vi "velosterpaser384.vi"(0 "roll":dbl=0.5000000000000001, 1 "pitch":dbl=-6.0, 2 "heading":dbl=1.2, 3 "dX":dbl=-0.009999999999999997, 4 "dY":dbl=1.287, 5 "dZ":dbl=1.6, 7 "Velodyne":T1(ring)=enum."Velodyne 64") -> (17 "pos_velo":dbl[](array[numeric]))   [LabVIEW 2015]
uses:
  G_LCM.vi
  G_SEN.vi
  <vilib>/Analysis/Matrix/Numeric/Conversions/Array To Matrix - RA2.vi
  <vilib>/Analysis/Matrix/Numeric/Multiply/Multiply - RM,RM.vi
  <vilib>/Analysis/Matrix/NI_Matrix.lvlib
panel:
  out "idx":i32[](array[numeric])
  out "Array":i32[](array[numeric])
  out "deleted portion":dbl[][](array[numeric])
  out "transposed array":dbl[][](array[numeric])
  out "o":dbl[](array[numeric])
  out "V":dbl[](array[numeric])
  out "R":dbl[](array[numeric])
  in  "PLOT":T1(ring)=enum."Velodyne 64"
  out "error out":errorcluster
  out "XY Graph 2":cluster{"X":dbl, "Y":dbl}[](graph)
  out "d":dbl[](array[numeric])
  in  "thresh":dbl
  out "i":u8[](array[numeric])
  out "Z":dbl[](array[numeric])
  out "Y":dbl[](array[numeric])
  out "X":dbl[](array[numeric])
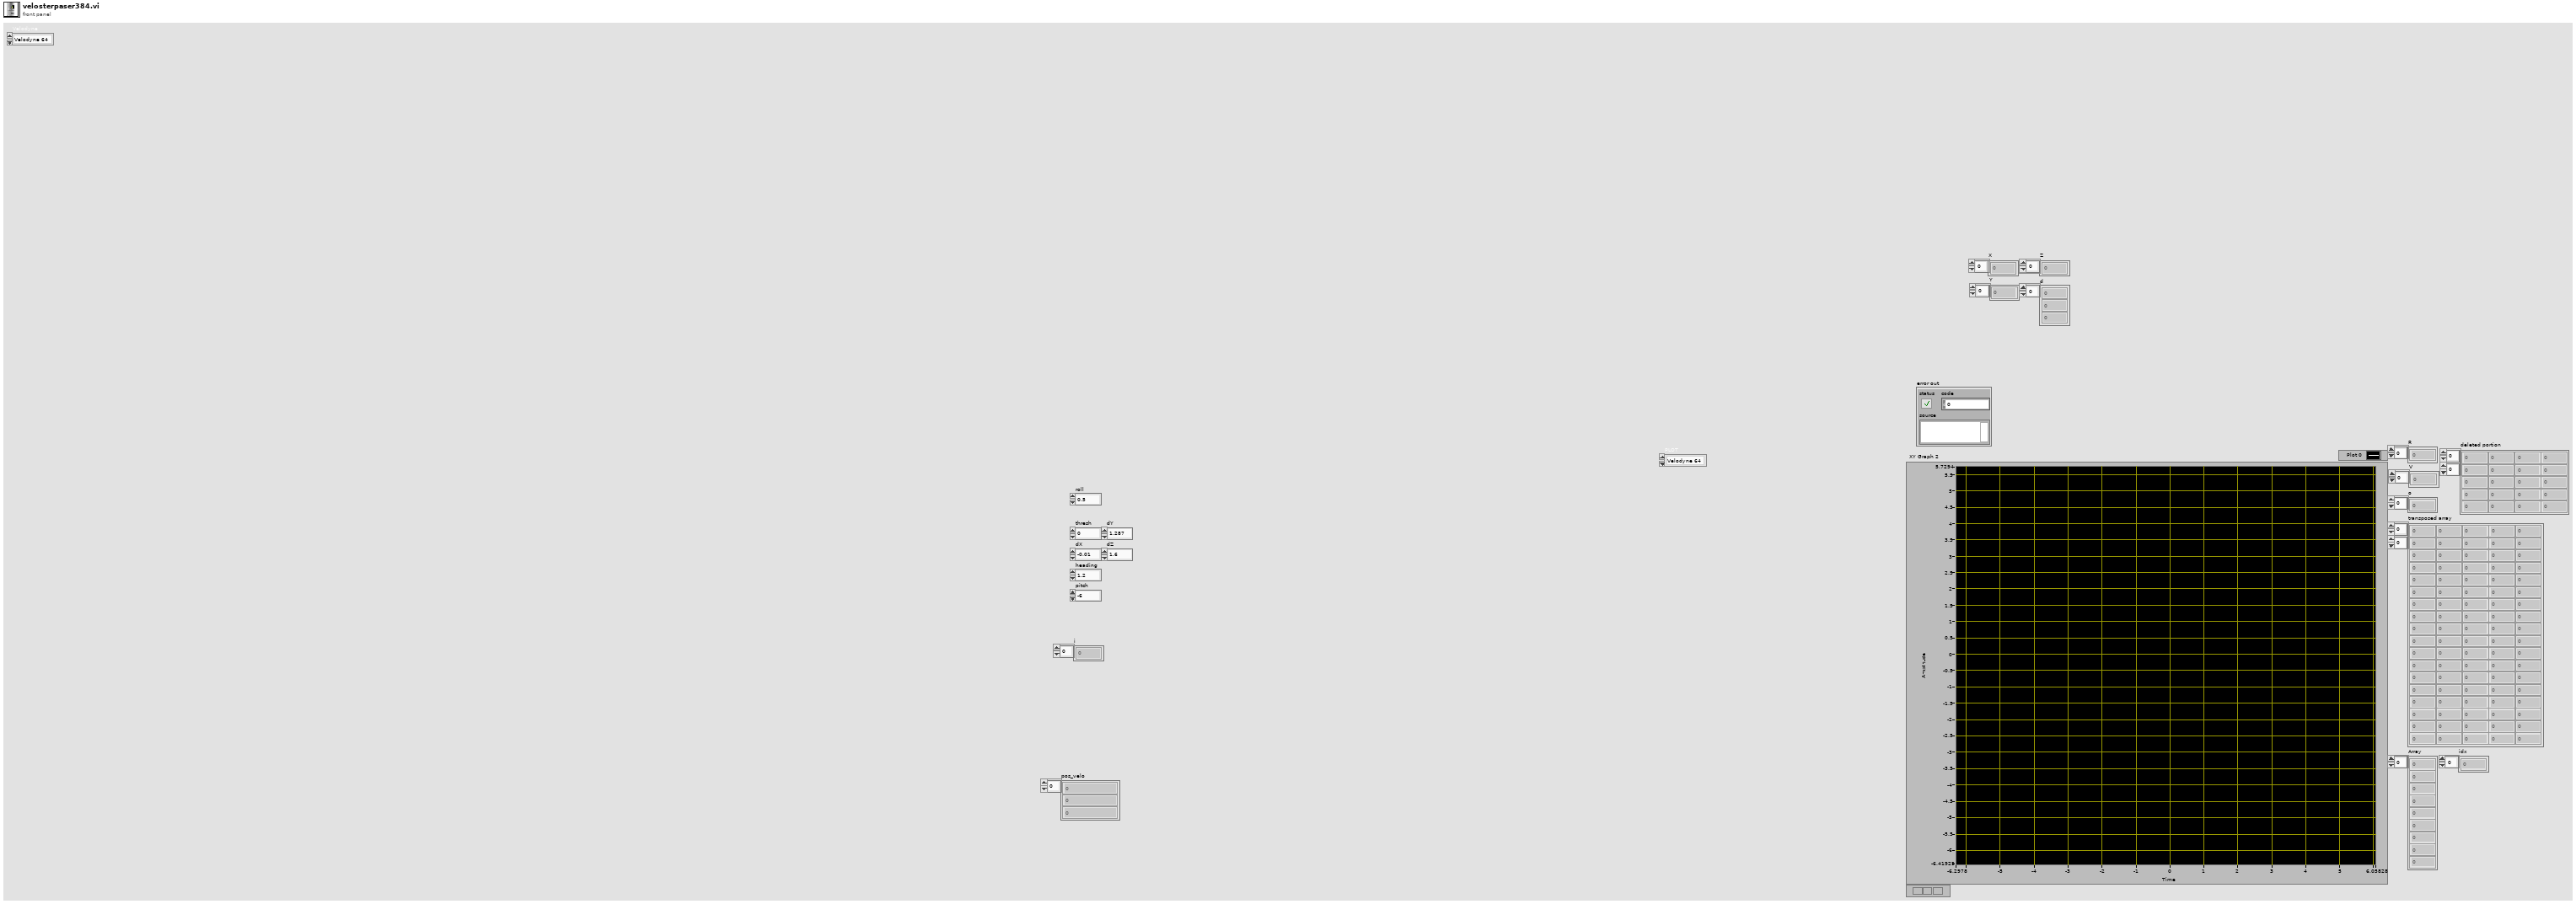
[diagram p1: front panel]
types:
  T1 = enum16{"Velodyne 16", "Velodyne 32", "Velodyne 64"}
  T2 = cluster{"hash":i64, "sys time":i64, "Timestamp":u32, "Rot_ang":dbl[], "Ver_ang":dbl[], "Dist":dbl[], "Ver_off":dbl[], "Intensity":u8[], "pos x":dbl, "pos y":dbl, "Heading":dbl}
  T3 = typedef "NI_Matrix.lvlib/RealMatrix.ctl" = dbl[][]
  T4 = cluster{i16, dbl, dbl, dbl, "Rotational position":dbl, "element":u8}[]
  T5 = cluster{dbl, i32, dbl, "Rotational position":dbl, dbl, "element":u8}[]
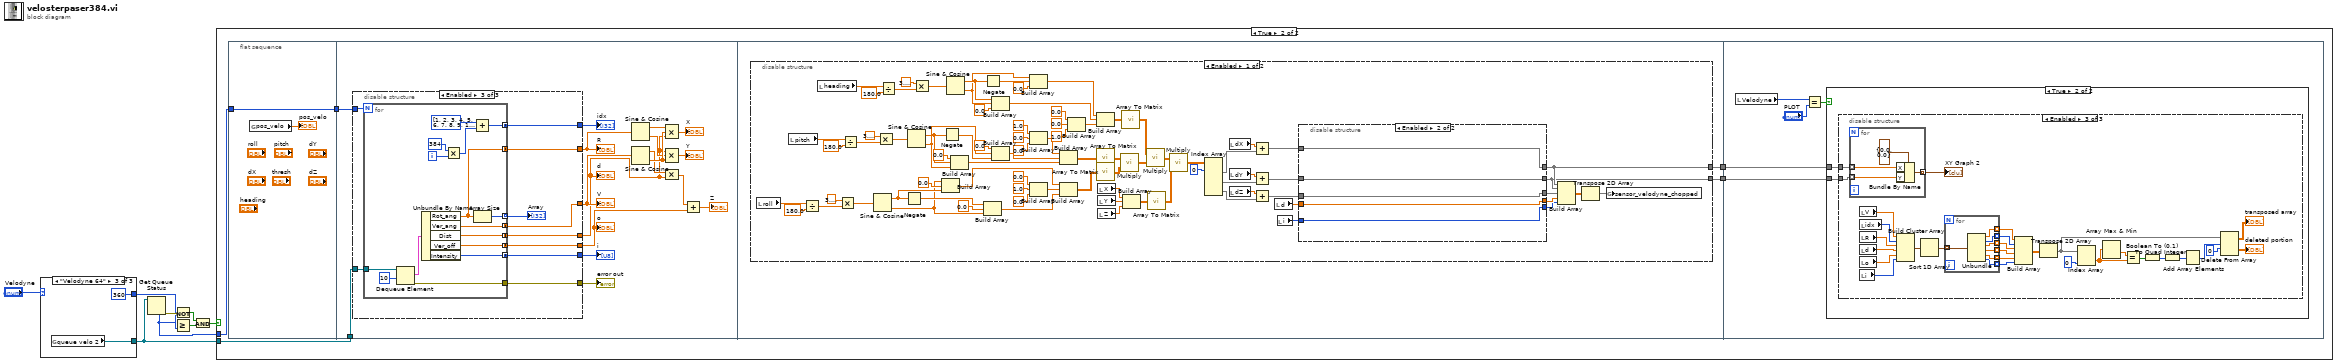
[diagram p0: block diagram]
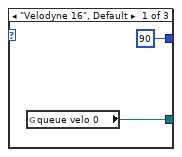
[diagram p2: hidden frame]
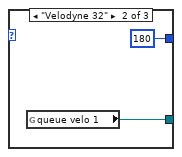
[diagram p3: hidden frame]
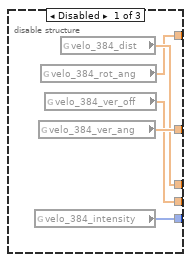
[diagram p5: hidden frame]
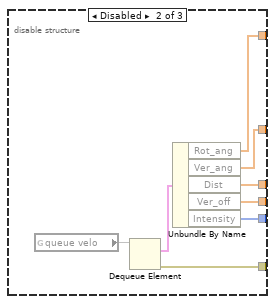
[diagram p6: hidden frame]
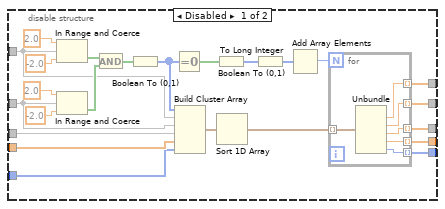
[diagram p7: hidden frame]
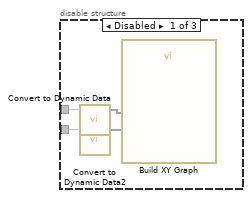
[diagram p10: hidden frame]
diagram:
  n1 = case shown="\"Velodyne 64\"" "Velodyne" {
    tunnel: [90 ("Numeric") 180 360 ("Numeric")] -> w5
    tunnel: [w9 w11 w13] -> w1
    frame "Velodyne 16", Default {
      n2 = global read "G_LCM.vi" "queue velo 0"() -> (w9:refnum<queue>)
    }
    frame "Velodyne 32" {
      n3 = global read "G_LCM.vi" "queue velo 1"() -> (w11:refnum<queue>)
    }
    frame "Velodyne 64" {
      n4 = global read "G_LCM.vi" "queue velo 2"() -> (w13:refnum<queue>)
    }
  }
  n5 = Get Queue Status(queue=w1) -> (error out=w7:errorcluster, # elements in queue=w2:i32)  [unwired: 2 in, 6 out]
  n6 = Not(x=w7) -> (.not. x?=w6:bool)
  n7 = Greater Or Equal?(x=w2, y=w5) -> (x >= y?=w8:bool)
  n8 = And(x=w6, y=w8) -> (x .and. y?=w4:bool)
  n9 = case shown="True" w4 {
    tunnel: w2 -> [_ w16]
    tunnel: w1 -> [_ w15]
    frame False {
    }
    frame True {
      n10 = flat-sequence {
        tunnel: [w20] -> w17
        tunnel: w16 -> [w20]
        tunnel: w17 -> [w24]
        tunnel: w15 -> [w23]
        tunnel: [w78] -> w19
        tunnel: [w77] -> w18
        tunnel: w19 -> [w199]
        tunnel: w18 -> [w198]
        frame #0 {
          n11 = global read "G_SEN.vi" "pos_velo"() -> (→"pos_velo":dbl[])
        }
        frame #1 {
          n12 = disable-structure shown="Enabled" {
            disable-tunnel: [w43 w49 w60] -> w38
            disable-tunnel: [w42 w47 w58] -> w32
            disable-tunnel: [w41 w46 w57] -> w28
            disable-tunnel: [w40 w48 w59] -> w27
            disable-tunnel: [w39 w50 w61] -> w26
            disable-tunnel: [_ w44 w56] -> w25
            disable-tunnel: w24 -> [_ _ w55]
            disable-tunnel: w23 -> [_ _ w54]
            disable-tunnel: [_ _ w52] -> w22
            frame Disabled {
              n13 = global read "G_SEN.vi" "velo_384_intensity"() -> (w41:u8[])
              n14 = global read "G_SEN.vi" "velo_384_ver_ang"() -> (w43:dbl[])
              n15 = global read "G_SEN.vi" "velo_384_rot_ang"() -> (w39:dbl[])
              n16 = global read "G_SEN.vi" "velo_384_ver_off"() -> (w42:dbl[])
              n17 = global read "G_SEN.vi" "velo_384_dist"() -> (w40:dbl[])
            }
            frame Disabled {
              n18 = global read "G_LCM.vi" "queue velo"() -> (w45)
              n19 = Dequeue Element(queue=w45) -> (element=w51:T2, error out=w44:errorcluster)  [unwired: 2 in, 2 out]
              n20 = Unbundle By Name(w51) -> ("Rot_ang"=w50:dbl[], "Ver_ang"=w49:dbl[], "Dist"=w48:dbl[], "Ver_off"=w47:dbl[], "Intensity"=w46:u8[])
            }
            frame Enabled {
              n21 = for {
                N: w55 -> [_]
                tunnel: w54 -> [w76]
                tunnel: [w68] -> w61 mode=concatenating
                tunnel: [w74] -> w60 mode=concatenating
                tunnel: [w73] -> w59 mode=concatenating
                tunnel: [w72] -> w58 mode=concatenating
                tunnel: [w71] -> w57 mode=concatenating
                tunnel: [w70] -> w56
                tunnel: [w67] -> w53 mode=indexing
                tunnel: [w62] -> w52 mode=concatenating
                i -> [w66]
                n22 = Dequeue Element(queue=w76, timeout in ms (-1)=10) -> (element=w75:T2, error out=w70:errorcluster)  [unwired: 1 in, 2 out]
                n23 = Unbundle By Name(w75) -> ("Rot_ang"=w68:dbl[], "Ver_ang"=w74:dbl[], "Dist"=w73:dbl[], "Ver_off"=w72:dbl[], "Intensity"=w71:u8[])
                n24 = Multiply(x=384, y=w66) -> (x*y=w64:i32)
                n25 = Add(x=i32[] [1, 2, 3, 4, 5, 6, 7, 8, 9, 10, 11, 12, 13, 14, 15, 16, 17, 18, 19, 20, 21, 22, 23, 24, 25, 26, 27, 28, 29, 30, 31, 32, 33, 34, 35, 36, 37, 38, 39, 40, 41, 42, 43, 44, 45, 46, 47, 48, 49, 50, 51, 52, 53, 54, 55, 56, 57, 58, 59, 60, 61, 62, 63, 64, 65, 66, 67, 68, 69, 70, 71, 72, 73, 74, 75, 76, 77, 78, 79, 80, 81, 82, 83, 84, 85, 86, 87, 88, 89, 90, 91, 92, 93, 94, 95, 96, 97, 98, 99, 100, 101, 102, 103, 104, 105, 106, 107, 108, 109, 110, 111, 112, 113, 114, 115, 116, 117, 118, 119, 120, 121, 122, 123, 124, 125, 126, 127, 128, 129, 130, 131, 132, 133, 134, 135, 136, 137, 138, 139, 140, 141, 142, 143, 144, 145, 146, 147, 148, 149, 150, 151, 152, 153, 154, 155, 156, 157, 158, 159, 160, 161, 162, 163, 164, 165, 166, 167, 168, 169, 170, 171, 172, 173, 174, 175, 176, 177, 178, 179, 180, 181, 182, 183, 184, 185, 186, 187, 188, 189, 190, 191, 192, 193, 194, 195, 196, 197, 198, 199, 200, 201, 202, 203, 204, 205, 206, 207, 208, 209, 210, 211, 212, 213, 214, 215, 216, 217, 218, 219, 220, 221, 222, 223, 224, 225, 226, 227, 228, 229, 230, 231, 232, 233, 234, 235, 236, 237, 238, 239, 240, 241, 242, 243, 244, 245, 246, 247, 248, 249, 250, 251, 252, 253, 254, 255, 256, 257, 258, 259, 260, 261, 262, 263, 264, 265, 266, 267, 268, 269, 270, 271, 272, 273, 274, 275, 276, 277, 278, 279, 280, 281, 282, 283, 284, 285, 286, 287, 288, 289, 290, 291, 292, 293, 294, 295, 296, 297, 298, 299, 300, 301, 302, 303, 304, 305, 306, 307, 308, 309, 310, 311, 312, 313, 314, 315, 316, 317, 318, 319, 320, 321, 322, 323, 324, 325, 326, 327, 328, 329, 330, 331, 332, 333, 334, 335, 336, 337, 338, 339, 340, 341, 342, 343, 344, 345, 346, 347, 348, 349, 350, 351, 352, 353, 354, 355, 356, 357, 358, 359, 360, 361, 362, 363, 364, 365, 366, 367, 368, 369, 370, 371, 372, 373, 374, 375, 376, 377, 378, 379, 380, 381, 382, 383, 384] ("x+1"), y=w64) -> (x+y=w62:i32[])
                n26 = Array Size(array=w68) -> (size(s)=w67:i32)
              }
              "Array" <- w53
            }
          }
          "d" <- w27
          "i" <- w28
          "error out" <- w25
          "R" <- w26
          "V" <- w38
          "o" <- w32
          "idx" <- w22
          n27 = Sine & Cosine(0:w26) -> (1:w36:dbl[], 2:w35:dbl[])
          n28 = Sine & Cosine(0:w38) -> (1:w34:dbl[], 2:w37:dbl[])
          n29 = Compound Arithmetic op=MULTIPLY(w36, w37, w27) -> (→"X":dbl[])
          n30 = Compound Arithmetic op=MULTIPLY(w27, w35, w37) -> (→"Y":dbl[])
          n31 = Compound Arithmetic op=MULTIPLY(w34, w27) -> (w33:dbl[])
          n32 = Add(x=w33, y=w32) -> (x+y=→"Z":dbl[])
        }
        frame #2 {
          n33 = disable-structure shown="Enabled" {
            disable-tunnel: [w80 _] -> w78
            disable-tunnel: [w79 _] -> w77
            frame Enabled {
              n34 = local read "roll"() -> (w92:dbl)
              n35 = local read "pitch"() -> (w101:dbl)
              n36 = Divide(x=w92, y=180.0) -> (x/y=w94:dbl)
              n37 = local read "heading"() -> (w96:dbl)
              n38 = Multiply(x=3.141592653589793, y=w94) -> (x*y=w90:dbl)
              n39 = Divide(x=w101, y=180.0) -> (x/y=w104:dbl)
              n40 = Sine & Cosine(0:w90) -> (1:w146:dbl, 2:w143:dbl)
              n41 = Multiply(x=3.141592653589793, y=w104) -> (x*y=w100:dbl)
              n42 = Divide(x=w96, y=180.0) -> (x/y=w97:dbl)
              n43 = Negate(x=w146) -> (-x=w145:dbl)
              n44 = Sine & Cosine(0:w100) -> (1:w130:dbl, 2:w133:dbl)
              n45 = Multiply(x=3.141592653589793, y=w97) -> (x*y=w95:dbl)
              n46 = Build Array(w143, 0.0 ("element"), w146) -> (w148:dbl[])
              n47 = Negate(x=w130) -> (-x=w132:dbl)
              n48 = Sine & Cosine(0:w95) -> (1:w127:dbl, 2:w125:dbl)
              n49 = Build Array(0.0 ("element"), w130, w133) -> (w129:dbl[])
              n50 = Build Array(w145, 0.0 ("element"), w143) -> (w142:dbl[])
              n51 = Negate(x=w127) -> (-x=w126:dbl)
              n52 = Build Array(w127, w125, 0.0 ("element")) -> (w128:dbl[])
              n53 = Build Array(0.0 ("element"), w133, w132) -> (w135:dbl[])
              n54 = Build Array(w125, w126, 0.0 ("element")) -> (w124:dbl[])
              n55 = Build Array(1.0 ("element"), 0.0 ("element"), 0.0 ("element")) -> (w136:dbl[])
              n56 = Build Array(0.0 ("element"), 1.0 ("element"), 0.0 ("element")) -> (w147:dbl[])
              n57 = Build Array(w136, w135, w129) -> (w140:dbl[][])
              n58 = Build Array(w148, w147, w142) -> (w141:dbl[][])
              n59 = Build Array(0.0 ("element"), 0.0 ("element"), 1.0 ("element")) -> (w119:dbl[])
              n60 = Build Array(w124, w128, w119) -> (w120:dbl[][])
              n61 = call-poly <vilib>:"Array To Matrix.vi"("Real 2D Array"=w140) -> ("Real Matrix"=w115:T3)
              n62 = call-poly <vilib>:"Array To Matrix.vi"("Real 2D Array"=w141) -> ("Real Matrix"=w116:T3)
              n63 = local read "X"() -> (w112:dbl[])
              n64 = local read "Y"() -> (w111:dbl[])
              n65 = local read "Z"() -> (w110:dbl[])
              n66 = call-poly <vilib>:"Multiply.vi"("Real Matrix B"=w116, "Real Matrix A"=w115) -> ("A * B"=w114:T3)
              n67 = call-poly <vilib>:"Array To Matrix.vi"("Real 2D Array"=w120) -> ("Real Matrix"=w113:T3)
              n68 = Build Array(w112, w111, w110) -> (w109:dbl[][])
              n69 = call-poly <vilib>:"Multiply.vi"("Real Matrix B"=w114, "Real Matrix A"=w113) -> ("A * B"=w108:T3)
              n70 = call-poly <vilib>:"Array To Matrix.vi"("Real 2D Array"=w109) -> ("Real Matrix"=w107:T3)
              n71 = call-poly <vilib>:"Multiply.vi"("Real Matrix B"=w107, "Real Matrix A"=w108) -> ("A * B"=w106:T3)
              n72 = Index Array(array=w106, index (row) #1=0 ("index (row)")) -> (element #1=w155:dbl[], element #2=w157:dbl[], element #3=w159:dbl[])  [unwired: 5 in]
              n73 = local read "dX"() -> (w154:dbl)
              n74 = local read "dY"() -> (w156:dbl)
              n75 = local read "dZ"() -> (w158:dbl)
              n76 = Add(x=w154, y=w155) -> (x+y=w88:dbl[])
              n77 = Add(x=w156, y=w157) -> (x+y=w85:dbl[])
              n78 = Add(x=w158, y=w159) -> (x+y=w153:dbl[])
              n79 = local read "d"() -> (w87:dbl[])
              n80 = local read "i"() -> (w86:u8[])
              n81 = disable-structure shown="Enabled" {
                disable-tunnel: w153 -> [w183 w192]
                disable-tunnel: w88 -> [w175 w194]
                disable-tunnel: w87 -> [w174 w191]
                disable-tunnel: w86 -> [w173 w190]
                disable-tunnel: [w167 w194] -> w80
                disable-tunnel: w85 -> [w166 w193]
                disable-tunnel: [w165 w193] -> w79
                disable-tunnel: [w164 w192] -> w84
                disable-tunnel: [w163 w191] -> w83
                disable-tunnel: [w162 w190] -> w82
                frame Disabled {
                  n82 = In Range and Coerce(upper limit=2.0, x=w175, lower limit=-2.0) -> (In Range?=w180:bool[])  [unwired: 1 out]
                  n83 = In Range and Coerce(upper limit=2.0, x=w166, lower limit=-2.0) -> (In Range?=w177:bool[])  [unwired: 1 out]
                  n84 = And(x=w180, y=w177) -> (x .and. y?=w176:bool[])
                  n85 = Boolean To (0,1)(Boolean=w176) -> (0, 1=w171:i16[])
                  n86 = Equal To 0?(x=w171) -> (x = 0?=w170:bool[])
                  n87 = Build Cluster Array(w171, w175, w166, w183, w174, w173) -> (w172:T4)
                  n88 = Boolean To (0,1)(Boolean=w170) -> (0, 1=w161:i16[])
                  n89 = Sort 1D Array(array=w172) -> (sorted array=w168:T4)
                  n90 = To Long Integer(number=w161) -> (32bit integer=w160:i32[])
                  n91 = Add Array Elements(numeric array=w160) -> (sum=w169:i32)
                  n92 = for {
                    N: w169 -> [_]
                    tunnel: w168 -> [w189] mode=indexing
                    tunnel: [w188] -> w167 mode=indexing
                    tunnel: [w187] -> w165 mode=indexing
                    tunnel: [w186] -> w164 mode=indexing
                    tunnel: [w185] -> w163 mode=indexing
                    tunnel: [w184] -> w162 mode=indexing
                    n93 = Unbundle(w189) -> (w188:dbl, w187:dbl, w186:dbl, "Rotational position"=w185:dbl, "element"=w184:u8)  [unwired: 1 out]
                  }
                }
                frame Enabled {
                }
              }
              n94 = Build Array(w80, w79, w84, w83, w82) -> (w89:dbl[][])
              n95 = Transpose 2D Array(2D array=w89) -> (transposed array=w81:dbl[][])
              n96 = global write "G_SEN.vi" "sensor_velodyne_chopped"(w81) -> ()
            }
            frame Disabled {
            }
          }
        }
        frame #3 {
          n97 = local read "Velodyne"() -> (w197:T1)
          n98 = Equal?(x=w197, y="PLOT") -> (x = y?=w195:bool)
          n99 = case shown="True" w195 {
            tunnel: w199 -> [_ w201]
            tunnel: w198 -> [_ w200]
            frame False {
            }
            frame True {
              n100 = disable-structure shown="Enabled" {
                disable-tunnel: w201 -> [w203 _ w233]
                disable-tunnel: w200 -> [w202 _ w232]
                frame Disabled {
                  n101 = call "Convert to Dynamic Data"("Array"=w203) -> ("Dynamic Data Type"=w205:dynamicdata)  [unwired: 3 in]
                  n102 = call "Convert to Dynamic Data2"("Array"=w202) -> ("Dynamic Data Type"=w204:dynamicdata)  [unwired: 3 in]
                  n103 = call "Build XY Graph"("Y Input"=w204, "X Input"=w205) -> ()  [unwired: 8 in, 2 out]
                }
                frame Disabled {
                }
                frame Enabled {
                  n104 = for {
                    tunnel: w233 -> [w244] mode=indexing
                    tunnel: w232 -> [w243] mode=indexing
                    tunnel: [w242] -> w234 mode=indexing
                    n105 = Bundle By Name(cluster=cluster{"X":dbl, "Y":dbl} {"X"=0.0, "Y"=0.0}, "X"=w244, "Y"=w243) -> (w242:cluster{"X":dbl, "Y":dbl})
                  }
                  "XY Graph 2" <- w234
                  n106 = local read "V"() -> (w208:dbl[])
                  n107 = local read "idx"() -> (w207:i32[])
                  n108 = local read "R"() -> (w231:dbl[])
                  n109 = local read "d"() -> (w230:dbl[])
                  n110 = local read "o"() -> (w212:dbl[])
                  n111 = local read "i"() -> (w211:u8[])
                  n112 = Build Cluster Array(w208, w207, w231, w230, w212, w211) -> (w229:T5)
                  n113 = Sort 1D Array(array=w229) -> (sorted array=w228:T5)
                  n114 = for {
                    tunnel: w228 -> [w241] mode=indexing
                    tunnel: [w240] -> w227 mode=indexing
                    tunnel: [w239] -> w226 mode=indexing
                    tunnel: [w238] -> w225 mode=indexing
                    tunnel: [w237] -> w210 mode=indexing
                    tunnel: [w236] -> w209 mode=indexing
                    tunnel: [w235] -> w206 mode=indexing
                    n115 = Unbundle(w241) -> (w240:dbl, w239:i32, w238:dbl, "Rotational position"=w237:dbl, w236:dbl, "element"=w235:u8)
                  }
                  n116 = Build Array(w227, w226, w225, w210, w209, w206) -> (w224:dbl[][])
                  n117 = Transpose 2D Array(2D array=w224) -> (transposed array=w217:dbl[][])
                  n118 = Index Array(array=w217, index (col)=0 ("disabled index (col)")) -> (element=w221:dbl[])  [unwired: 1 in]
                  n119 = Array Max & Min(array=w221) -> (min value=w222:dbl)  [unwired: 3 out]
                  n120 = Equal?(x=w222, y=w221) -> (x = y?=w220:bool[])
                  n121 = Boolean To (0,1)(Boolean=w220) -> (0, 1=w219:i16[])
                  n122 = To Quad Integer(1:w219) -> (0:w218:i64[])
                  n123 = Add Array Elements(numeric array=w218) -> (sum=w216:i64)
                  n124 = Delete From Array(array=w217, length=w216, index (row)=0) -> (deleted portion=→"deleted portion":dbl[][], array with subset deleted=→"transposed array":dbl[][])  [unwired: 1 in]
                }
              }
            }
          }
        }
      }
    }
  }
